vi "matchRelevantVIsvn.vi"(10 "logEntry":string, 11 "associatedVIs":string[](array[string])) -> (1 "found":bool, 3 "relevantPath":string)   [LabVIEW 2021]
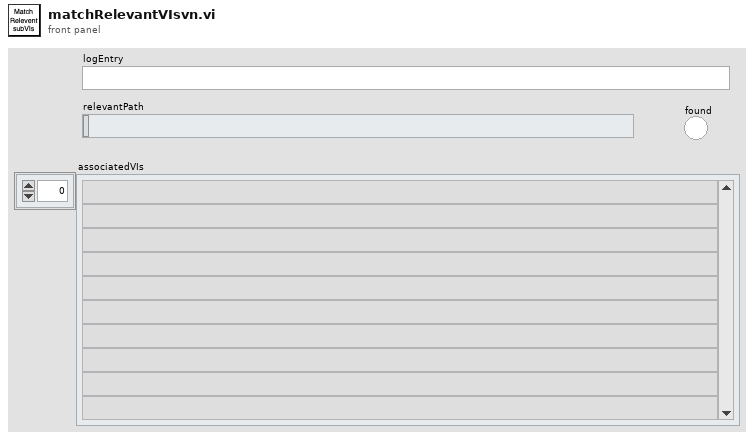
[diagram p1: front panel]
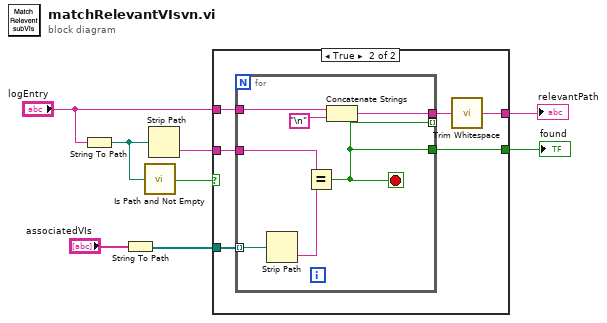
[diagram p0: block diagram]
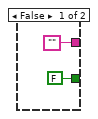
[diagram p2: hidden frame]
diagram:
  n1 = String To Path(string="logEntry") -> (path=w2:path)
  n2 = String To Path(string="associatedVIs") -> (path=w6:path[])
  n3 = call <vilib>:"Is Path and Not Empty.vi"("path"=w2) -> ("Is Path and Not Empty?"=w1:bool)  [unwired: 4 in]
  n4 = Strip Path(path=w2) -> (name=w5:string)  [unwired: 1 out]
  n5 = case shown="True" w1 {
    tunnel: "logEntry" -> [_ w15]
    tunnel: w6 -> [_ w14]
    tunnel: w5 -> [_ w13]
    tunnel: [FALSE w12] -> w4
    tunnel: ["" w11] -> w3
    frame False {
    }
    frame True {
      n6 = for {
        tunnel: [w22] -> w16 if=w17
        tunnel: w15 -> [w23]
        tunnel: w14 -> [w20] mode=indexing
        tunnel: w13 -> [w19]
        tunnel: [w17] -> _ mode=indexing
        tunnel: [w17] -> w12
        stop <- w17 stop-if-true
        n7 = Strip Path(path=w20) -> (name=w18:string)  [unwired: 1 out]
        n8 = Equal?(x=w19, y=w18) -> (x = y?=w17:bool)
        n9 = Concatenate Strings(w23, "\n") -> (w22:string)
      }
      n10 = call <vilib>:"Trim Whitespace.vi"("string"=w16) -> ("trimmed string"=w11:string)  [unwired: 1 in]
    }
  }
  "relevantPath" <- w3
  "found" <- w4
